vi "Add Emp.vi"(8 "error in (no error)":errorcluster caption="错误输入（无错误）", 10 "迭代器.lvlib:雇员.lvclass":refnum<class "雇员.lvclass">, 11 "雇员名录管理 输入":refnum<class "雇员名录管理.lvclass"> caption="DNL_LabVIEW Object in") -> (0 "error out":errorcluster caption="错误输出", 3 "雇员名录管理 输出":refnum<class "雇员名录管理.lvclass"> caption="DNL_LabVIEW Object out")   [LabVIEW 2011, in "迭代器.lvlib" / "雇员名录管理.lvclass"]
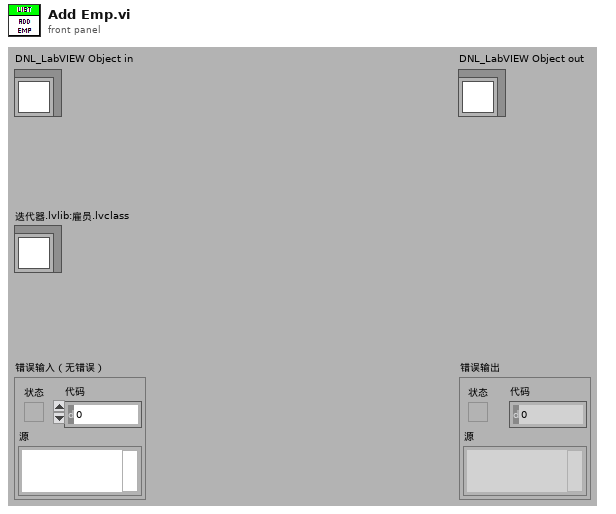
[diagram p1: front panel]
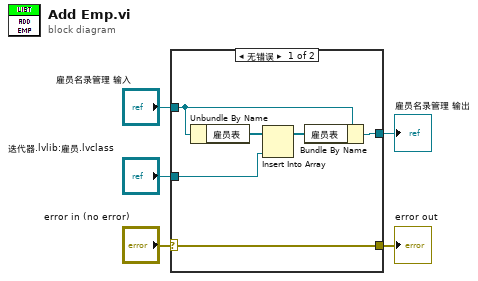
[diagram p0: block diagram]
diagram:
  n1 = case shown="无错误" "error in (no error)" {
    selector: "error in (no error)" -> [w11 w13]
    tunnel: [w11 w13] -> w4
    tunnel: [w9 w12] -> w2
    tunnel: "雇员名录管理 输入" -> [w10 w12]
    tunnel: "迭代器.lvlib:雇员.lvclass" -> [w7 _]
    frame No Error {
      n2 = Unbundle By Name(w10) -> ("雇员表"=w8:refnum<class "雇员.lvclass">[])
      n3 = Insert Into Array(array=w8, new element=w7) -> (w6:refnum<class "雇员.lvclass">[])  [unwired: 1 in]
      n4 = Bundle By Name(cluster=w10, "雇员表"=w6) -> (w9:refnum<class "雇员名录管理.lvclass">)
    }
    frame Error {
    }
  }
  "error out" <- w4
  "雇员名录管理 输出" <- w2
